vi "var_stop.vi"() -> ()   [LabVIEW 2014]
panel:
  out "system stop":bool
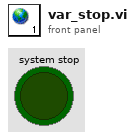
[diagram p1: front panel]
diagram:
